vi "Conditional Open Connection.vi"(8 "error in (no error)":errorcluster, 11 "TCP Network Connection in":refnum<k5>) -> (0 "error out":errorcluster, 3 "TCP Network Connection out":refnum<k5>)   [LabVIEW 2020]
doc: "This software is licensed for use under the “MIT License\"\nCopyright (c) 2019 Scott Hannahs, sth@alum.mit.edu\n\nPermission is hereby granted, free of charge, to any person obtaining a copy of this software and associated documentation files (the \"Software\"), to deal in the Software without restriction, including without limitation the rights to use, copy, modify, merge, publish, distribute, sublicense, and/or sell copies of the Software, and to permit persons to whom the Software is furnished to do so, subject to the following conditions: The above copyright notice and this permission notice shall be included in all copies or substantial portions of the Software.\n\nTHE SOFTWARE IS PROVIDED \"AS IS\", WITHOUT WARRANTY OF ANY KIND, EXPRESS OR IMPLIED, INCLUDING BUT NOT LIMITED TO THE WARRANTIES OF MERCHANTABILITY, FITNESS FOR A PARTICULAR PURPOSE AND NONINFRINGEMENT. IN NO EVENT SHALL THE AUTHORS OR COPYRIGHT HOLDERS BE LIABLE FOR ANY CLAIM, DAMAGES OR OTHER LIABILITY, WHETHER IN AN ACTION OF CONTRACT, TORT OR OTHERWISE, ARISING FROM, OUT OF OR IN CONNECTION WITH THE SOFTWARE OR THE USE OR OTHER DEALINGS IN THE SOFTWARE."
uses:
  SubVIs/Interlock 32T Net Client Globals.vi
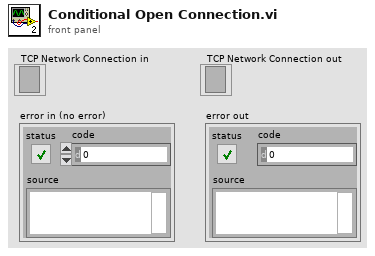
[diagram p1: front panel]
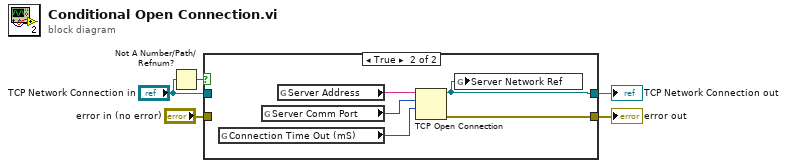
[diagram p0: block diagram]
diagram:
  n1 = Not A Number/Path/Refnum?(number/path/refnum="TCP Network Connection in") -> (NaN/Path/Refnum?=w1:bool)
  n2 = case shown="True" w1 {
    tunnel: [w7 w11] -> w5
    tunnel: "TCP Network Connection in" -> [w7 _]
    tunnel: [w6 w12] -> w4
    tunnel: "error in (no error)" -> [w6 _]
    frame False {
    }
    frame True {
      n3 = global read "Interlock 32T Net Client Globals.vi" "Connection Time Out (mS)"() -> (w8:i32)
      n4 = global read "Interlock 32T Net Client Globals.vi" "Server Comm Port"() -> (w9:u16)
      n5 = global read "Interlock 32T Net Client Globals.vi" "Server Address"() -> (w10:string)
      n6 = TCP Open Connection(address=w10, remote port or service name=w9, timeout ms (60000)=w8) -> (connection ID=w11:refnum<k5>, error out=w12:errorcluster)  [unwired: 2 in]
      n7 = global write "Interlock 32T Net Client Globals.vi" "Server Network Ref"(w11) -> ()
    }
  }
  "TCP Network Connection out" <- w5
  "error out" <- w4
